vi "RTS Find Enabled Station For TempHumidity.vi"(8 "Error In":errorcluster, 11 "All Door Opener Ctrl":T4 {"Station 8"."Station Slide"."Chamber 1-1"."Start Time" format="%<%X\n%x>T"; "Station 8"."Station Slide"."Chamber 1-1"."End Time" format="%<%X\n%x>T"; "Station 8"."Station Slide"."Time Count (s)" format="%.2f"; "Station 8"."Station Cab"."Chamber 1-1"."Start Time" format="%<%X\n%x>T"; "Station 8"."Station Cab"."Chamber 1-1"."End Time" format="%<%X\n%x>T"; "Station 8"."Station Cab"."Time Count (s)" format="%.2f"; "Station 8"."Station Freezer"."Chamber 1-1"."Start Time" format="%<%X\n%x>T"; "Station 8"."Station Freezer"."Chamber 1-1"."End Time" format="%<%X\n%x>T"; "Station 8"."Station Freezer"."Time Count (s)" format="%.2f"; "Station 7"."Station Slide"."Chamber 1-1"."Start Time" format="%<%X\n%x>T"; "Station 7"."Station Slide"."Chamber 1-1"."End Time" format="%<%X\n%x>T"; "Station 7"."Station Slide"."Time Count (s)" format="%.2f"; "Station 7"."Station Cab"."Chamber 1-1"."Start Time" format="%<%X\n%x>T"; "Station 7"."Station Cab"."Chamber 1-1"."End Time" format="%<%X\n%x>T"; "Station 7"."Station Cab"."Time Count (s)" format="%.2f"; "Station 7"."Station Freezer"."Chamber 1-1"."Start Time" format="%<%X\n%x>T"; "Station 7"."Station Freezer"."Chamber 1-1"."End Time" format="%<%X\n%x>T"; "Station 7"."Station Freezer"."Time Count (s)" format="%.2f"; "Station 6"."Station Slide"."Chamber 1-1"."Start Time" format="%<%X\n%x>T"; "Station 6"."Station Slide"."Chamber 1-1"."End Time" format="%<%X\n%x>T"; "Station 6"."Station Slide"."Time Count (s)" format="%.2f"; "Station 6"."Station Cab"."Chamber 1-1"."Start Time" format="%<%X\n%x>T"; "Station 6"."Station Cab"."Chamber 1-1"."End Time" format="%<%X\n%x>T"; "Station 6"."Station Cab"."Time Count (s)" format="%.2f"; "Station 6"."Station Freezer"."Chamber 1-1"."Start Time" format="%<%X\n%x>T"; "Station 6"."Station Freezer"."Chamber 1-1"."End Time" format="%<%X\n%x>T"; "Station 6"."Station Freezer"."Time Count (s)" format="%.2f"; "Station 5"."Station Slide"."Chamber 1-1"."Start Time" format="%<%X\n%x>T"; "Station 5"."Station Slide"."Chamber 1-1"."End Time" format="%<%X\n%x>T"; "Station 5"."Station Slide"."Time Count (s)" format="%.2f"; "Station 5"."Station Cab"."Chamber 1-1"."Start Time" format="%<%X\n%x>T"; "Station 5"."Station Cab"."Chamber 1-1"."End Time" format="%<%X\n%x>T"; "Station 5"."Station Cab"."Time Count (s)" format="%.2f"; "Station 5"."Station Freezer"."Chamber 1-1"."Start Time" format="%<%X\n%x>T"; "Station 5"."Station Freezer"."Chamber 1-1"."End Time" format="%<%X\n%x>T"; "Station 5"."Station Freezer"."Time Count (s)" format="%.2f"; "Station 4"."Station Slide"."Chamber 1-1"."Start Time" format="%<%X\n%x>T"; "Station 4"."Station Slide"."Chamber 1-1"."End Time" format="%<%X\n%x>T"; "Station 4"."Station Slide"."Time Count (s)" format="%.2f"; "Station 4"."Station Cab"."Chamber 1-1"."Start Time" format="%<%X\n%x>T"; "Station 4"."Station Cab"."Chamber 1-1"."End Time" format="%<%X\n%x>T"; "Station 4"."Station Cab"."Time Count (s)" format="%.2f"; "Station 4"."Station Freezer"."Chamber 1-1"."Start Time" format="%<%X\n%x>T"; "Station 4"."Station Freezer"."Chamber 1-1"."End Time" format="%<%X\n%x>T"; "Station 4"."Station Freezer"."Time Count (s)" format="%.2f"; "Station 3"."Station Slide"."Chamber 1-1"."Start Time" format="%<%X\n%x>T"; "Station 3"."Station Slide"."Chamber 1-1"."End Time" format="%<%X\n%x>T"; "Station 3"."Station Slide"."Time Count (s)" format="%.2f"; "Station 3"."Station Cab"."Chamber 1-1"."Start Time" format="%<%X\n%x>T"; "Station 3"."Station Cab"."Chamber 1-1"."End Time" format="%<%X\n%x>T"; "Station 3"."Station Cab"."Time Count (s)" format="%.2f"; "Station 3"."Station Freezer"."Chamber 1-1"."Start Time" format="%<%X\n%x>T"; "Station 3"."Station Freezer"."Chamber 1-1"."End Time" format="%<%X\n%x>T"; "Station 3"."Station Freezer"."Time Count (s)" format="%.2f"; "Station 2"."Station Slide"."Chamber 1-1"."Start Time" format="%<%X\n%x>T"; "Station 2"."Station Slide"."Chamber 1-1"."End Time" format="%<%X\n%x>T"; "Station 2"."Station Slide"."Time Count (s)" format="%.2f"; "Station 2"."Station Cab"."Chamber 1-1"."Start Time" format="%<%X\n%x>T"; "Station 2"."Station Cab"."Chamber 1-1"."End Time" format="%<%X\n%x>T"; "Station 2"."Station Cab"."Time Count (s)" format="%.2f"; "Station 2"."Station Freezer"."Chamber 1-1"."Start Time" format="%<%X\n%x>T"; "Station 2"."Station Freezer"."Chamber 1-1"."End Time" format="%<%X\n%x>T"; "Station 2"."Station Freezer"."Time Count (s)" format="%.2f"; "Station 1"."Station Slide"."Chamber 1-1"."Start Time" format="%<%X\n%x>T"; "Station 1"."Station Slide"."Chamber 1-1"."End Time" format="%<%X\n%x>T"; "Station 1"."Station Slide"."Time Count (s)" format="%.2f"; "Station 1"."Station Cab"."Chamber 1-1"."Start Time" format="%<%X\n%x>T"; "Station 1"."Station Cab"."Chamber 1-1"."End Time" format="%<%X\n%x>T"; "Station 1"."Station Cab"."Time Count (s)" format="%.2f"; "Station 1"."Station Freezer"."Chamber 1-1"."Start Time" format="%<%X\n%x>T"; "Station 1"."Station Freezer"."Chamber 1-1"."End Time" format="%<%X\n%x>T"; "Station 1"."Station Freezer"."Time Count (s)" format="%.2f"}) -> (0 "Error Out":errorcluster, 1 "Index":i32, 2 "Set Chamber Conditions":bool, 3 "Chamber 1-1":T1 {"Start Time" format="%<%X\n%x>T"; "End Time" format="%<%X\n%x>T"})   [LabVIEW 2016]
uses:
  Type Definitions/RTS All Station Door Opener Ctrl.ctl
  Type Definitions/RTS Station Relay Ops.ctl
  Type Definitions/RTS Door Opener Indicator.ctl
  Type Definitions/RTS Door Ops Client.ctl
  Type Definitions/RTS Door Opening Schedule.ctl
  Type Definitions/RTS Door Ops Sequence.ctl
panel:
  # "Chamber Conditions:"
  # "Chamber Conditions:"
  # "Chamber Conditions:"
  # "Chamber Conditions:"
  # "Chamber Conditions:"
  # "Chamber Conditions:"
  # "Chamber Conditions:"
  # "Chamber Conditions:"
  # "Chamber Conditions:"
  # "Chamber Conditions:"
  # "Chamber Conditions:"
  # "Chamber Conditions:"
  # "Chamber Conditions:"
  # "Chamber Conditions:"
  # "Chamber Conditions:"
  # "Chamber Conditions:"
  # "Chamber Conditions:"
  # "Chamber Conditions:"
  # "Chamber Conditions:"
  # "Chamber Conditions:"
  # "Chamber Conditions:"
  # "Chamber Conditions:"
  # "Chamber Conditions:"
  # "Chamber Conditions:"
  # "Chamber Conditions:"
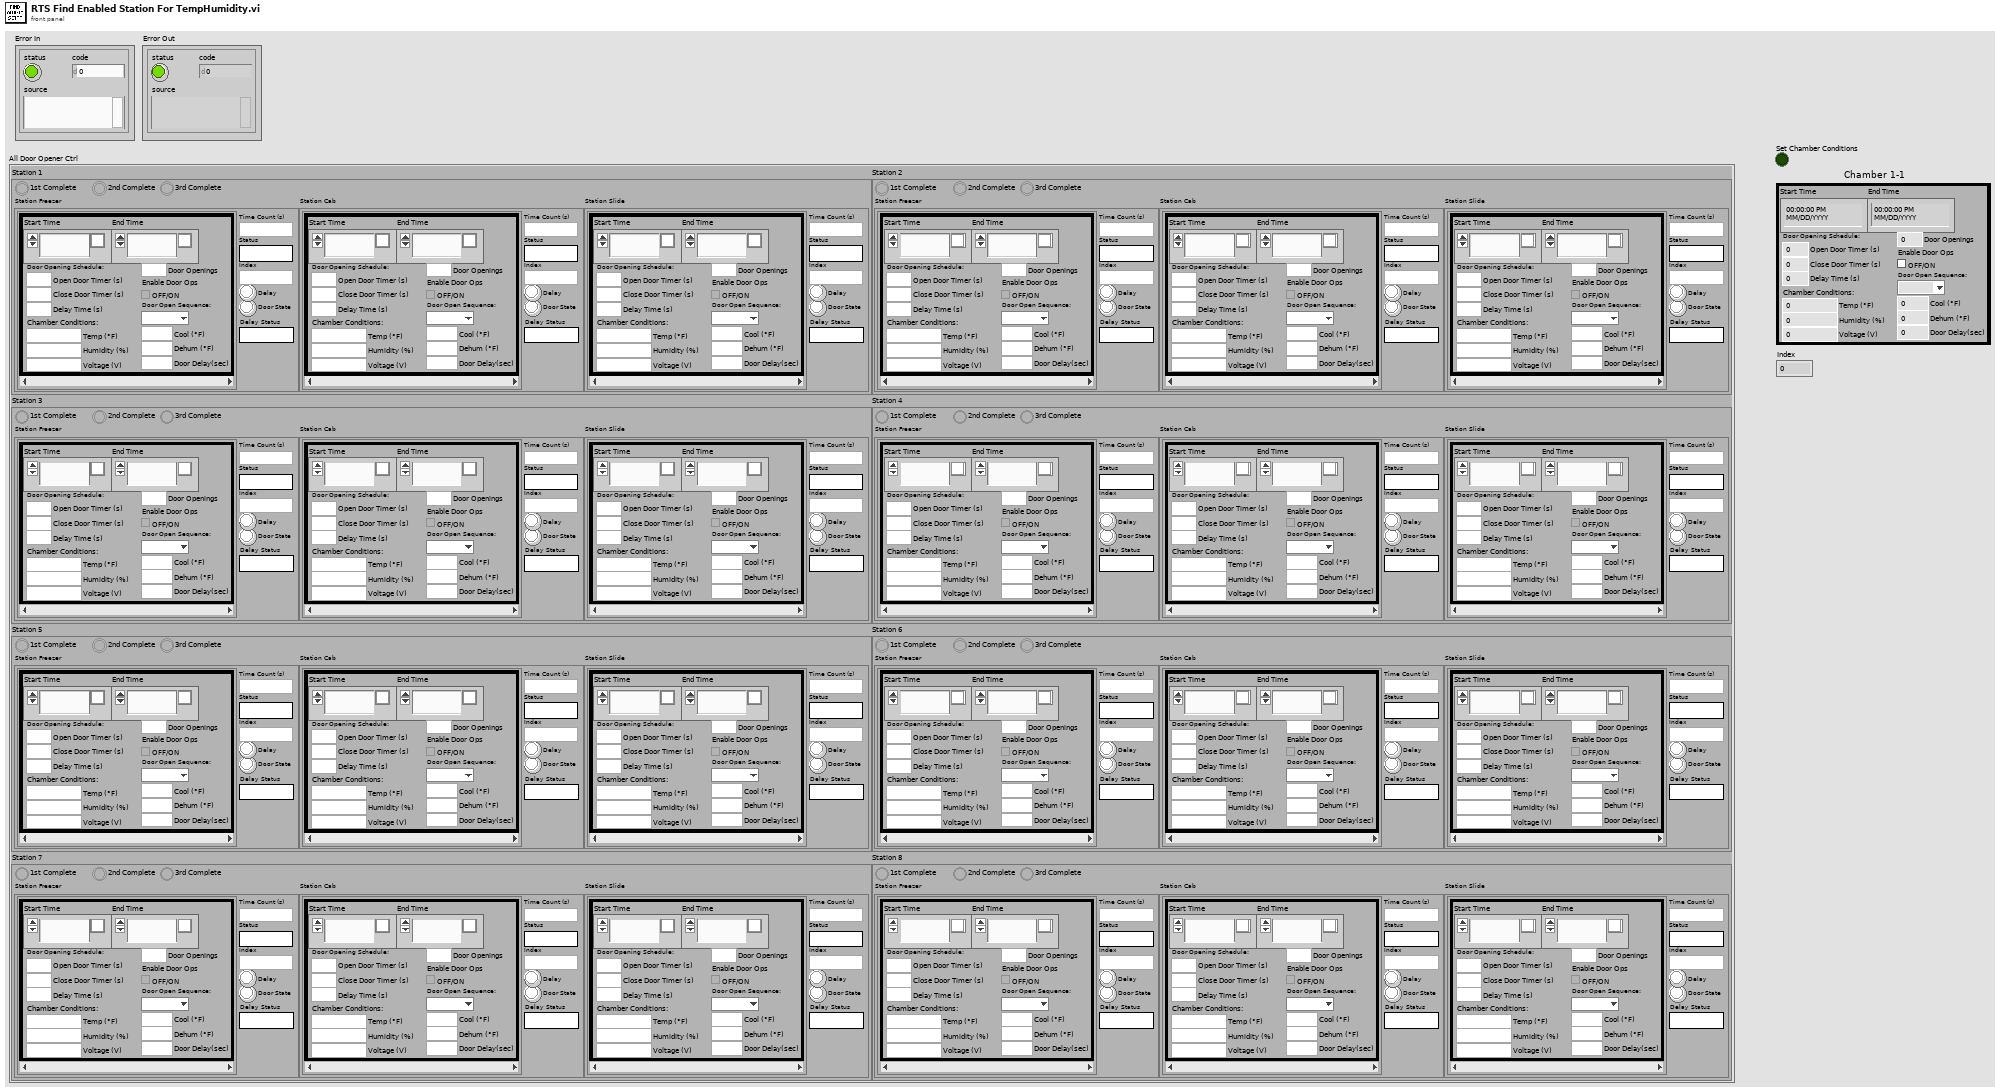
[diagram p1: front panel]
types:
  T1 = typedef "RTS Door Ops Client.ctl" = cluster{"End Time":timestamp, "Start Time":timestamp, "Door Opening Schedule:":T2, "Enable Door Ops":bool, "Door Openings":u32, "Temp (°F)":dbl, "Humidity (%)":dbl, "Voltage (V)":dbl, "Door Open Sequence:":T3, "Door Delay(sec)":dbl, "Dehum (°F)":dbl, "Cool (°F)":dbl}
  T2 = typedef "RTS Door Opening Schedule.ctl" = cluster{"Open Door Timer (s)":dbl, "Delay Time (s)":dbl, "Close Door Timer (s)":dbl}
  T3 = typedef "RTS Door Ops Sequence.ctl" = enum16{"", "1st", "2nd", "3rd"}
  T4 = typedef "RTS All Station Door Opener Ctrl.ctl" = cluster{"Station 1":T5, "Station 2":T5, "Station 3":T5, "Station 4":T5, "Station 5":T5, "Station 6":T5, "Station 7":T5, "Station 8":T5}
  T5 = typedef "RTS Station Relay Ops.ctl" = cluster{"Station Freezer":T6, "Station Cab":T6, "Station Slide":T6, "1st Complete":bool, "2nd Complete":bool, "3rd Complete":bool}
  T6 = typedef "RTS Door Opener Indicator.ctl" = cluster{"Time Count (s)":dbl, "Status":string, "Door State":bool, "Delay":bool, "Chamber 1-1":T1[], "Index":i32, "Delay Status":string}
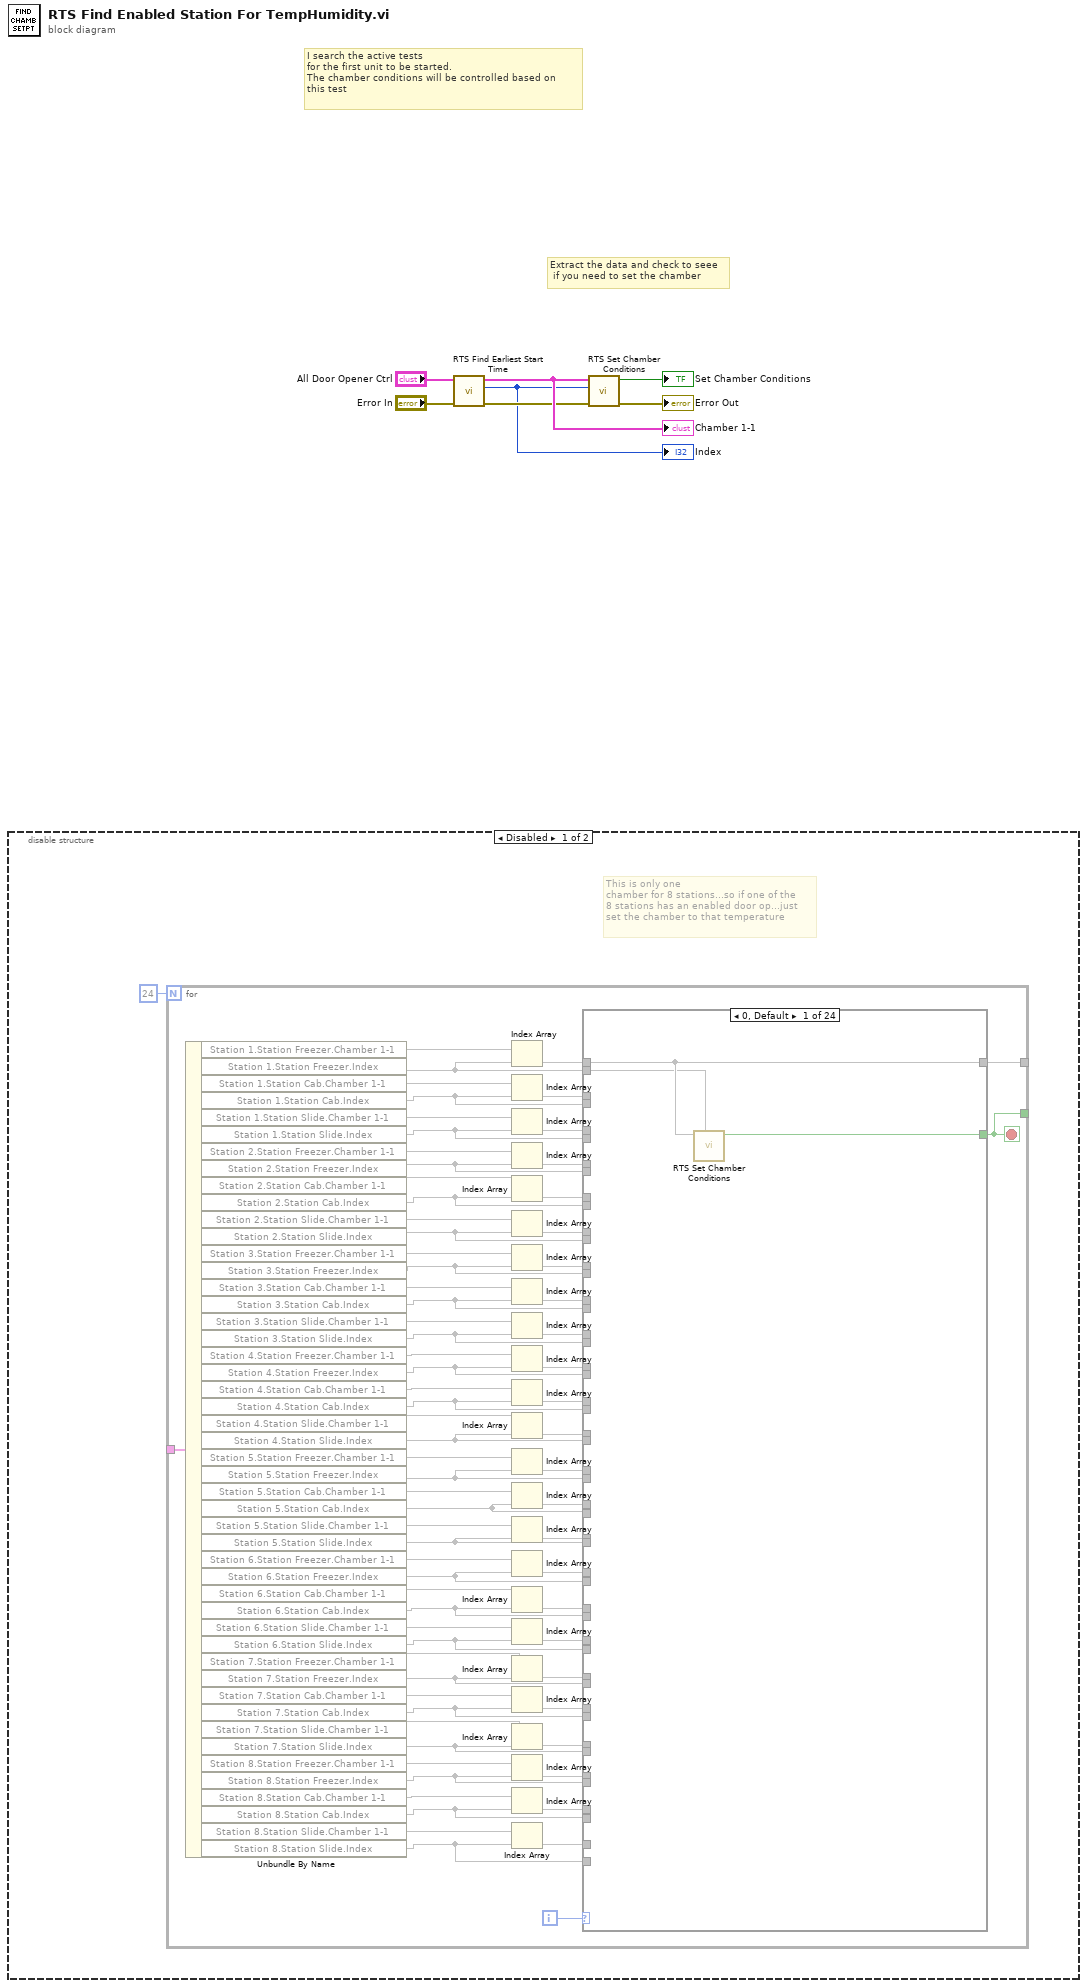
[diagram p0: block diagram]
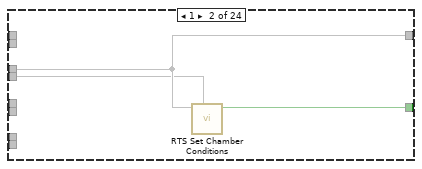
[diagram p2: hidden frame]
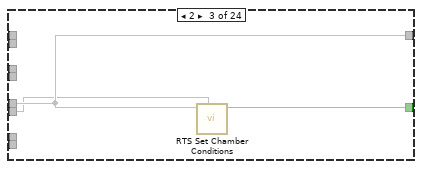
[diagram p3: hidden frame]
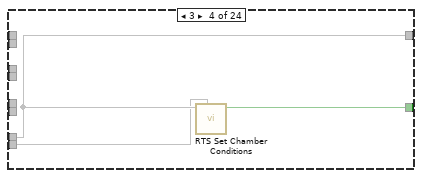
[diagram p4: hidden frame]
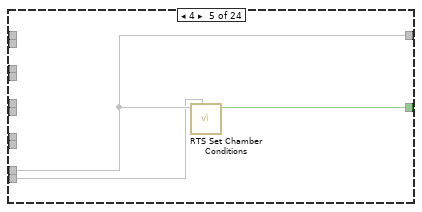
[diagram p5: hidden frame]
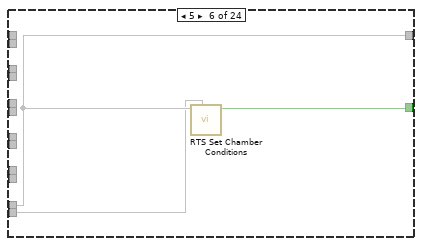
[diagram p6: hidden frame]
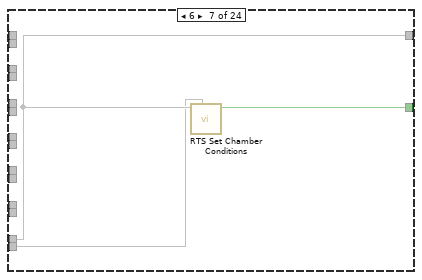
[diagram p7: hidden frame]
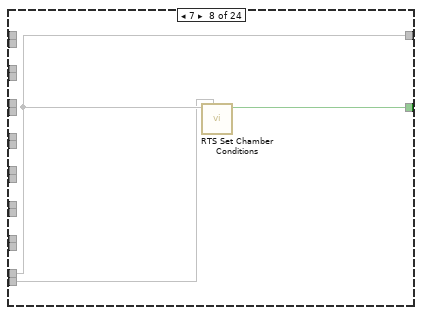
[diagram p8: hidden frame]
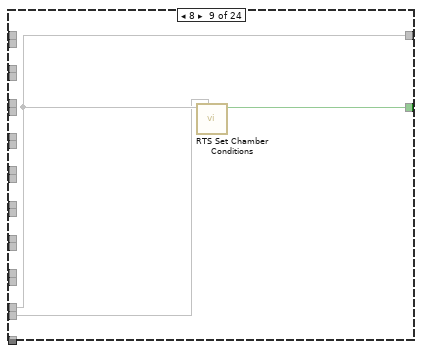
[diagram p9: hidden frame]
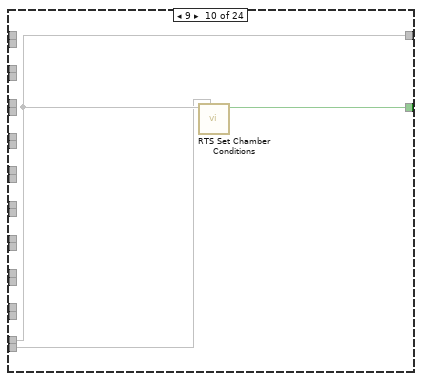
[diagram p10: hidden frame]
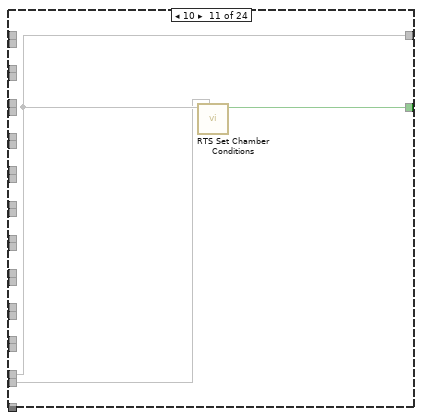
[diagram p11: hidden frame]
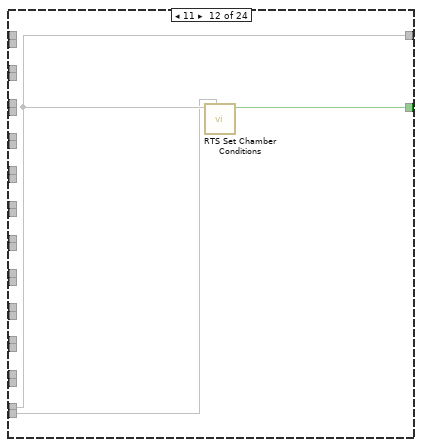
[diagram p12: hidden frame]
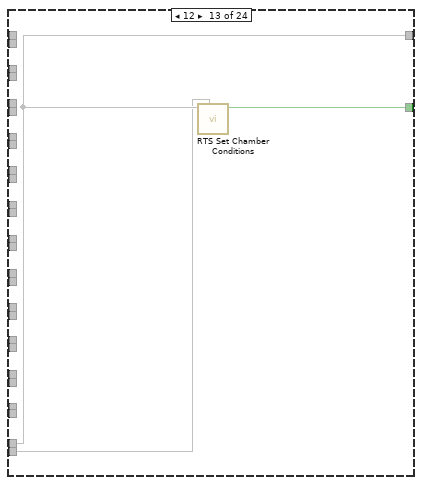
[diagram p13: hidden frame]
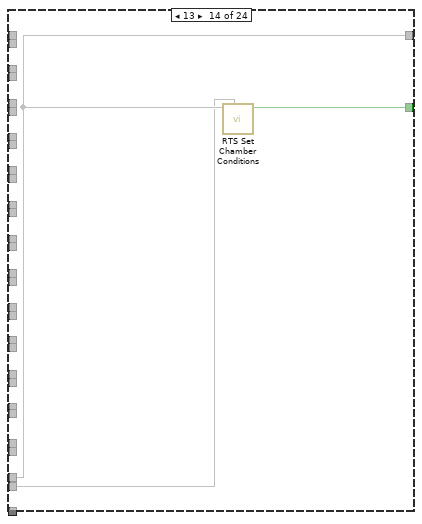
[diagram p14: hidden frame]
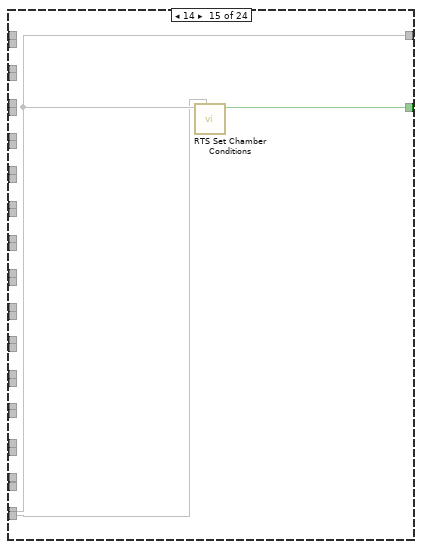
[diagram p15: hidden frame]
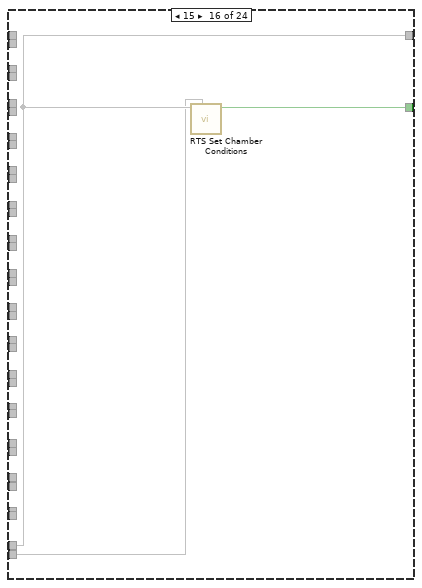
[diagram p16: hidden frame]
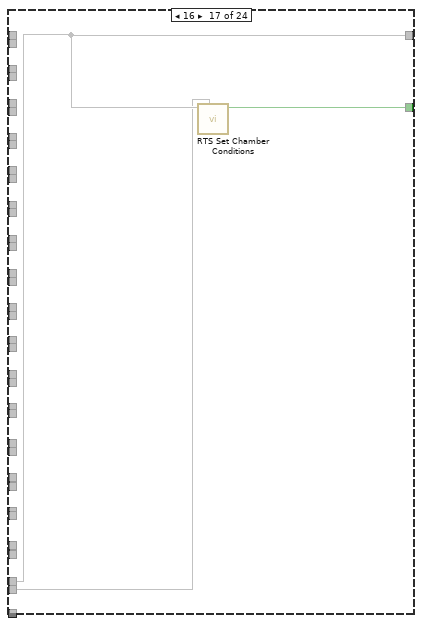
[diagram p17: hidden frame]
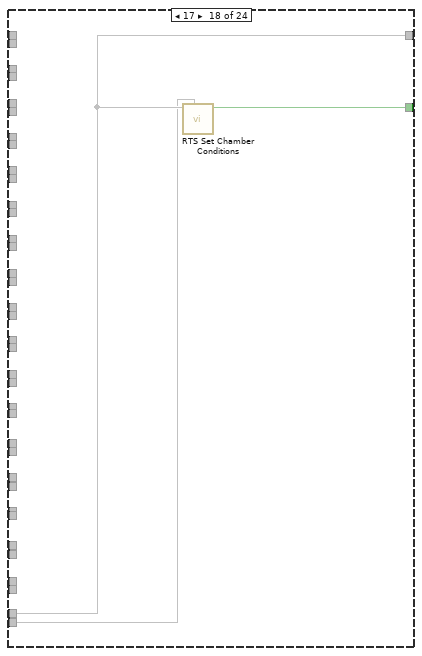
[diagram p18: hidden frame]
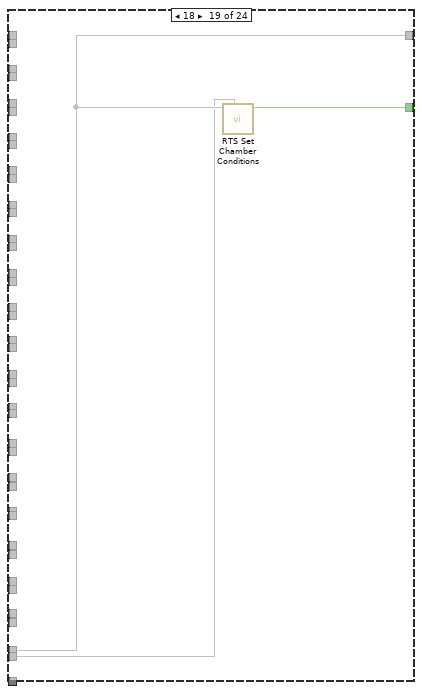
[diagram p19: hidden frame]
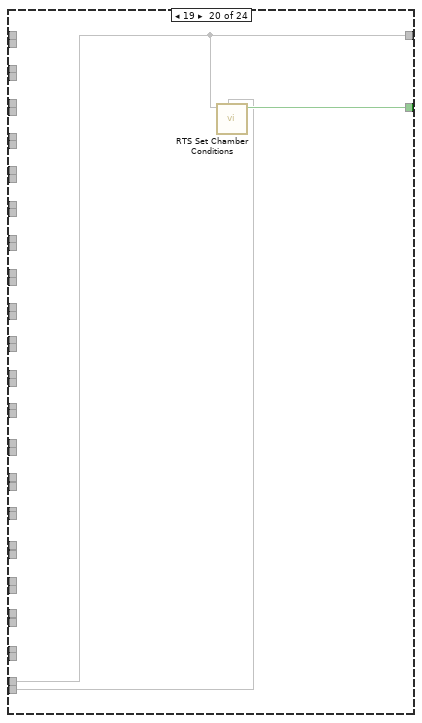
[diagram p20: hidden frame]
diagram:
  # "Extract the data and check to seee\n if you need to set the chamber"
  # "I search the active tests \nfor the first unit to be started.\nThe chamber conditions will be controlled based on\nthis test"
  n1 = disable-structure shown="Disabled" {
    frame Disabled {
      # "This is only one \nchamber for 8 stations...so if one of the \n8 stations has an enabled door op...just\nset the chamber to that temperature"
      n2 = for {
        N: 24 -> [_]
        tunnel: _ -> [w84]
        tunnel: [w79] -> _
        tunnel: [w9] -> _
        i -> [w10]
        stop <- w9 stop-if-true
        n3 = Unbundle By Name(w84) -> ("Station 1.Station Freezer.Chamber 1-1"=w83, "Station 1.Station Freezer.Index"=w34, "Station 1.Station Cab.Chamber 1-1"=w82, "Station 1.Station Cab.Index"=w32, "Station 1.Station Slide.Chamber 1-1"=w81, "Station 1.Station Slide.Index"=w31, "Station 2.Station Freezer.Chamber 1-1"=w76, "Station 2.Station Freezer.Index"=w30, "Station 2.Station Cab.Chamber 1-1"=w75, "Station 2.Station Cab.Index"=w33, "Station 2.Station Slide.Chamber 1-1"=w74, "Station 2.Station Slide.Index"=w29, "Station 3.Station Freezer.Chamber 1-1"=w73, "Station 3.Station Freezer.Index"=w28, "Station 3.Station Cab.Chamber 1-1"=w72, "Station 3.Station Cab.Index"=w27, "Station 3.Station Slide.Chamber 1-1"=w71, "Station 3.Station Slide.Index"=w26, "Station 4.Station Freezer.Chamber 1-1"=w70, "Station 4.Station Freezer.Index"=w25, "Station 4.Station Cab.Chamber 1-1"=w69, "Station 4.Station Cab.Index"=w24, "Station 4.Station Slide.Chamber 1-1"=w68, "Station 4.Station Slide.Index"=w23, "Station 5.Station Freezer.Chamber 1-1"=w67, "Station 5.Station Freezer.Index"=w22, "Station 5.Station Cab.Chamber 1-1"=w66, "Station 5.Station Cab.Index"=w21, "Station 5.Station Slide.Chamber 1-1"=w65, "Station 5.Station Slide.Index"=w20, "Station 6.Station Freezer.Chamber 1-1"=w64, "Station 6.Station Freezer.Index"=w19, "Station 6.Station Cab.Chamber 1-1"=w63, "Station 6.Station Cab.Index"=w18, "Station 6.Station Slide.Chamber 1-1"=w62, "Station 6.Station Slide.Index"=w17, "Station 7.Station Freezer.Chamber 1-1"=w61, "Station 7.Station Freezer.Index"=w16, "Station 7.Station Cab.Chamber 1-1"=w60, "Station 7.Station Cab.Index"=w15, "Station 7.Station Slide.Chamber 1-1"=w59, "Station 7.Station Slide.Index"=w14, "Station 8.Station Freezer.Chamber 1-1"=w58, "Station 8.Station Freezer.Index"=w13, "Station 8.Station Cab.Chamber 1-1"=w57, "Station 8.Station Cab.Index"=w12, "Station 8.Station Slide.Chamber 1-1"=w56, "Station 8.Station Slide.Index"=w11)
        n4 = Index Array(array=w83, index=w34) -> (element=w80)
        n5 = Index Array(array=w82, index=w32) -> (element=w78)
        n6 = Index Array(array=w81, index=w31) -> (element=w77)
        n7 = Index Array(array=w76, index=w30) -> (element=w55)
        n8 = Index Array(array=w75, index=w33) -> (element=w54)
        n9 = Index Array(array=w74, index=w29) -> (element=w53)
        n10 = Index Array(array=w73, index=w28) -> (element=w52)
        n11 = Index Array(array=w72, index=w27) -> (element=w51)
        n12 = Index Array(array=w71, index=w26) -> (element=w50)
        n13 = Index Array(array=w70, index=w25) -> (element=w49)
        n14 = Index Array(array=w69, index=w24) -> (element=w48)
        n15 = Index Array(array=w68, index=w23) -> (element=w47)
        n16 = Index Array(array=w67, index=w22) -> (element=w46)
        n17 = Index Array(array=w66, index=w21) -> (element=w45)
        n18 = Index Array(array=w65, index=w20) -> (element=w44)
        n19 = Index Array(array=w64, index=w19) -> (element=w43)
        n20 = Index Array(array=w63, index=w18) -> (element=w42)
        n21 = Index Array(array=w62, index=w17) -> (element=w41)
        n22 = Index Array(array=w61, index=w16) -> (element=w40)
        n23 = Index Array(array=w60, index=w15) -> (element=w39)
        n24 = Index Array(array=w59, index=w14) -> (element=w38)
        n25 = Index Array(array=w58, index=w13) -> (element=w37)
        n26 = Index Array(array=w57, index=w12) -> (element=w36)
        n27 = Index Array(array=w56, index=w11) -> (element=w35)
        n28 = case shown="0, Default" w10 {
          tunnel: w80 -> [w87 _ _ _ _ _ _ _ _ _ _ _ _ _ _ _ _ _ _ _ _ _ _ _]
          tunnel: [w87 w90 w93 w96 w99 w102 w105 w108 w111 w114 w117 w120 w122 w126 w129 w132 w135 w138 w141 w144 w147 w150 w153 w156] -> w79
          tunnel: [w86 w89 w92 w95 w98 w101 w104 w107 w110 w113 w116 w119 w123 w125 w128 w131 w134 w137 w140 w143 w146 w149 w152 w155] -> w9
          tunnel: w78 -> [_ w90 _ _ _ _ _ _ _ _ _ _ _ _ _ _ _ _ _ _ _ _ _ _]
          tunnel: w77 -> [_ _ w93 _ _ _ _ _ _ _ _ _ _ _ _ _ _ _ _ _ _ _ _ _]
          tunnel: w55 -> [_ _ _ w96 _ _ _ _ _ _ _ _ _ _ _ _ _ _ _ _ _ _ _ _]
          tunnel: w54 -> [_ _ _ _ w99 _ _ _ _ _ _ _ _ _ _ _ _ _ _ _ _ _ _ _]
          tunnel: w53 -> [_ _ _ _ _ w102 _ _ _ _ _ _ _ _ _ _ _ _ _ _ _ _ _ _]
          tunnel: w52 -> [_ _ _ _ _ _ w105 _ _ _ _ _ _ _ _ _ _ _ _ _ _ _ _ _]
          tunnel: w51 -> [_ _ _ _ _ _ _ w108 _ _ _ _ _ _ _ _ _ _ _ _ _ _ _ _]
          tunnel: w50 -> [_ _ _ _ _ _ _ _ w111 _ _ _ _ _ _ _ _ _ _ _ _ _ _ _]
          tunnel: w49 -> [_ _ _ _ _ _ _ _ _ w114 _ _ _ _ _ _ _ _ _ _ _ _ _ _]
          tunnel: w48 -> [_ _ _ _ _ _ _ _ _ _ w117 _ _ _ _ _ _ _ _ _ _ _ _ _]
          tunnel: w47 -> [_ _ _ _ _ _ _ _ _ _ _ w120 _ _ _ _ _ _ _ _ _ _ _ _]
          tunnel: w46 -> [_ _ _ _ _ _ _ _ _ _ _ _ w122 _ _ _ _ _ _ _ _ _ _ _]
          tunnel: w45 -> [_ _ _ _ _ _ _ _ _ _ _ _ _ w126 _ _ _ _ _ _ _ _ _ _]
          tunnel: w44 -> [_ _ _ _ _ _ _ _ _ _ _ _ _ _ w129 _ _ _ _ _ _ _ _ _]
          tunnel: w43 -> [_ _ _ _ _ _ _ _ _ _ _ _ _ _ _ w132 _ _ _ _ _ _ _ _]
          tunnel: w42 -> [_ _ _ _ _ _ _ _ _ _ _ _ _ _ _ _ w135 _ _ _ _ _ _ _]
          tunnel: w41 -> [_ _ _ _ _ _ _ _ _ _ _ _ _ _ _ _ _ w138 _ _ _ _ _ _]
          tunnel: w40 -> [_ _ _ _ _ _ _ _ _ _ _ _ _ _ _ _ _ _ w141 _ _ _ _ _]
          tunnel: w39 -> [_ _ _ _ _ _ _ _ _ _ _ _ _ _ _ _ _ _ _ w144 _ _ _ _]
          tunnel: w38 -> [_ _ _ _ _ _ _ _ _ _ _ _ _ _ _ _ _ _ _ _ w147 _ _ _]
          tunnel: w37 -> [_ _ _ _ _ _ _ _ _ _ _ _ _ _ _ _ _ _ _ _ _ w150 _ _]
          tunnel: w36 -> [_ _ _ _ _ _ _ _ _ _ _ _ _ _ _ _ _ _ _ _ _ _ w153 _]
          tunnel: w35 -> [_ _ _ _ _ _ _ _ _ _ _ _ _ _ _ _ _ _ _ _ _ _ _ w156]
          tunnel: w34 -> [w85 _ _ _ _ _ _ _ _ _ _ _ _ _ _ _ _ _ _ _ _ _ _ _]
          tunnel: w33 -> [_ _ _ _ w97 _ _ _ _ _ _ _ _ _ _ _ _ _ _ _ _ _ _ _]
          tunnel: w32 -> [_ w88 _ _ _ _ _ _ _ _ _ _ _ _ _ _ _ _ _ _ _ _ _ _]
          tunnel: w31 -> [_ _ w91 _ _ _ _ _ _ _ _ _ _ _ _ _ _ _ _ _ _ _ _ _]
          tunnel: w30 -> [_ _ _ w94 _ _ _ _ _ _ _ _ _ _ _ _ _ _ _ _ _ _ _ _]
          tunnel: w29 -> [_ _ _ _ _ w100 _ _ _ _ _ _ _ _ _ _ _ _ _ _ _ _ _ _]
          tunnel: w28 -> [_ _ _ _ _ _ w103 _ _ _ _ _ _ _ _ _ _ _ _ _ _ _ _ _]
          tunnel: w27 -> [_ _ _ _ _ _ _ w106 _ _ _ _ _ _ _ _ _ _ _ _ _ _ _ _]
          tunnel: w26 -> [_ _ _ _ _ _ _ _ w109 _ _ _ _ _ _ _ _ _ _ _ _ _ _ _]
          tunnel: w25 -> [_ _ _ _ _ _ _ _ _ w112 _ _ _ _ _ _ _ _ _ _ _ _ _ _]
          tunnel: w24 -> [_ _ _ _ _ _ _ _ _ _ w115 _ _ _ _ _ _ _ _ _ _ _ _ _]
          tunnel: w23 -> [_ _ _ _ _ _ _ _ _ _ _ w118 _ _ _ _ _ _ _ _ _ _ _ _]
          tunnel: w22 -> [_ _ _ _ _ _ _ _ _ _ _ _ w121 _ _ _ _ _ _ _ _ _ _ _]
          tunnel: w21 -> [_ _ _ _ _ _ _ _ _ _ _ _ _ w124 _ _ _ _ _ _ _ _ _ _]
          tunnel: w20 -> [_ _ _ _ _ _ _ _ _ _ _ _ _ _ w127 _ _ _ _ _ _ _ _ _]
          tunnel: w19 -> [_ _ _ _ _ _ _ _ _ _ _ _ _ _ _ w130 _ _ _ _ _ _ _ _]
          tunnel: w18 -> [_ _ _ _ _ _ _ _ _ _ _ _ _ _ _ _ w133 _ _ _ _ _ _ _]
          tunnel: w17 -> [_ _ _ _ _ _ _ _ _ _ _ _ _ _ _ _ _ w136 _ _ _ _ _ _]
          tunnel: w16 -> [_ _ _ _ _ _ _ _ _ _ _ _ _ _ _ _ _ _ w139 _ _ _ _ _]
          tunnel: w15 -> [_ _ _ _ _ _ _ _ _ _ _ _ _ _ _ _ _ _ _ w142 _ _ _ _]
          tunnel: w14 -> [_ _ _ _ _ _ _ _ _ _ _ _ _ _ _ _ _ _ _ _ w145 _ _ _]
          tunnel: w13 -> [_ _ _ _ _ _ _ _ _ _ _ _ _ _ _ _ _ _ _ _ _ w148 _ _]
          tunnel: w12 -> [_ _ _ _ _ _ _ _ _ _ _ _ _ _ _ _ _ _ _ _ _ _ w151 _]
          tunnel: w11 -> [_ _ _ _ _ _ _ _ _ _ _ _ _ _ _ _ _ _ _ _ _ _ _ w154]
          frame 0, Default {
            n29 = call "RTS Set Chamber Conditions.vi"(7:w85, "Chamber 1-1"=w87) -> ("Send Chamber Conditions"=w86:bool)  [unwired: 8 in, 1 out]
          }
          frame 1 {
            n30 = call "RTS Set Chamber Conditions.vi"(7:w88, "Chamber 1-1"=w90) -> ("Send Chamber Conditions"=w89:bool)  [unwired: 8 in, 1 out]
          }
          frame 2 {
            n31 = call "RTS Set Chamber Conditions.vi"(7:w91, "Chamber 1-1"=w93) -> ("Send Chamber Conditions"=w92:bool)  [unwired: 8 in, 1 out]
          }
          frame 3 {
            n32 = call "RTS Set Chamber Conditions.vi"(7:w94, "Chamber 1-1"=w96) -> ("Send Chamber Conditions"=w95:bool)  [unwired: 8 in, 1 out]
          }
          frame 4 {
            n33 = call "RTS Set Chamber Conditions.vi"(7:w97, "Chamber 1-1"=w99) -> ("Send Chamber Conditions"=w98:bool)  [unwired: 8 in, 1 out]
          }
          frame 5 {
            n34 = call "RTS Set Chamber Conditions.vi"(7:w100, "Chamber 1-1"=w102) -> ("Send Chamber Conditions"=w101:bool)  [unwired: 8 in, 1 out]
          }
          frame 6 {
            n35 = call "RTS Set Chamber Conditions.vi"(7:w103, "Chamber 1-1"=w105) -> ("Send Chamber Conditions"=w104:bool)  [unwired: 8 in, 1 out]
          }
          frame 7 {
            n36 = call "RTS Set Chamber Conditions.vi"(7:w106, "Chamber 1-1"=w108) -> ("Send Chamber Conditions"=w107:bool)  [unwired: 8 in, 1 out]
          }
          frame 8 {
            n37 = call "RTS Set Chamber Conditions.vi"(7:w109, "Chamber 1-1"=w111) -> ("Send Chamber Conditions"=w110:bool)  [unwired: 8 in, 1 out]
          }
          frame 9 {
            n38 = call "RTS Set Chamber Conditions.vi"(7:w112, "Chamber 1-1"=w114) -> ("Send Chamber Conditions"=w113:bool)  [unwired: 8 in, 1 out]
          }
          frame 10 {
            n39 = call "RTS Set Chamber Conditions.vi"(7:w115, "Chamber 1-1"=w117) -> ("Send Chamber Conditions"=w116:bool)  [unwired: 8 in, 1 out]
          }
          frame 11 {
            n40 = call "RTS Set Chamber Conditions.vi"(7:w118, "Chamber 1-1"=w120) -> ("Send Chamber Conditions"=w119:bool)  [unwired: 8 in, 1 out]
          }
          frame 12 {
            n41 = call "RTS Set Chamber Conditions.vi"(7:w121, "Chamber 1-1"=w122) -> ("Send Chamber Conditions"=w123:bool)  [unwired: 8 in, 1 out]
          }
          frame 13 {
            n42 = call "RTS Set Chamber Conditions.vi"(7:w124, "Chamber 1-1"=w126) -> ("Send Chamber Conditions"=w125:bool)  [unwired: 8 in, 1 out]
          }
          frame 14 {
            n43 = call "RTS Set Chamber Conditions.vi"(7:w127, "Chamber 1-1"=w129) -> ("Send Chamber Conditions"=w128:bool)  [unwired: 8 in, 1 out]
          }
          frame 15 {
            n44 = call "RTS Set Chamber Conditions.vi"(7:w130, "Chamber 1-1"=w132) -> ("Send Chamber Conditions"=w131:bool)  [unwired: 8 in, 1 out]
          }
          frame 16 {
            n45 = call "RTS Set Chamber Conditions.vi"(7:w133, "Chamber 1-1"=w135) -> ("Send Chamber Conditions"=w134:bool)  [unwired: 8 in, 1 out]
          }
          frame 17 {
            n46 = call "RTS Set Chamber Conditions.vi"(7:w136, "Chamber 1-1"=w138) -> ("Send Chamber Conditions"=w137:bool)  [unwired: 8 in, 1 out]
          }
          frame 18 {
            n47 = call "RTS Set Chamber Conditions.vi"(7:w139, "Chamber 1-1"=w141) -> ("Send Chamber Conditions"=w140:bool)  [unwired: 8 in, 1 out]
          }
          frame 19 {
            n48 = call "RTS Set Chamber Conditions.vi"(7:w142, "Chamber 1-1"=w144) -> ("Send Chamber Conditions"=w143:bool)  [unwired: 8 in, 1 out]
          }
          frame 20 {
            n49 = call "RTS Set Chamber Conditions.vi"(7:w145, "Chamber 1-1"=w147) -> ("Send Chamber Conditions"=w146:bool)  [unwired: 8 in, 1 out]
          }
          frame 21 {
            n50 = call "RTS Set Chamber Conditions.vi"(7:w148, "Chamber 1-1"=w150) -> ("Send Chamber Conditions"=w149:bool)  [unwired: 8 in, 1 out]
          }
          frame 22 {
            n51 = call "RTS Set Chamber Conditions.vi"(7:w151, "Chamber 1-1"=w153) -> ("Send Chamber Conditions"=w152:bool)  [unwired: 8 in, 1 out]
          }
          frame 23 {
            n52 = call "RTS Set Chamber Conditions.vi"(7:w154, "Chamber 1-1"=w156) -> ("Send Chamber Conditions"=w155:bool)  [unwired: 8 in, 1 out]
          }
        }
      }
    }
    frame Enabled {
    }
  }
  n53 = call "RTS Find Earliest Start Time.vi"("Error In"="Error In", "All Door Opener Ctrl"="All Door Opener Ctrl") -> ("Error Out"=w5:errorcluster, "Index"=w1:i32, "Chamber 1-1"=w6:T1)  [unwired: 7 in]
  "Chamber 1-1" <- w6
  "Index" <- w1
  n54 = call "RTS Set Chamber Conditions.vi"("Error In"=w5, "Index"=w1, "Chamber 1-1"=w6) -> ("Error Out"=→"Error Out":errorcluster, "Send Chamber Conditions"=→"Set Chamber Conditions":bool)  [unwired: 7 in]
